vi "Handle Error.vi"(8 "error in (no error)":errorcluster, 11 "Guardian in":refnum<class "Guardian.lvclass">) -> (0 "error out":errorcluster, 2 "stop actor?":bool=TRUE, 3 "Guardian out":refnum<class "Guardian.lvclass">)   [LabVIEW 2026, in "TALOS.lvlib" / "Guardian.lvlib" / "Guardian.lvclass"]
doc: "This VI will process every error generated by a Guardian. If it is possible to solve it, log it in locale and not pass it to the Ancestor: otherwise, let it go, the Ancestor will try to do the same and, ultimately, it will push the error to the Error Manager of the Distributed System."
uses:
  Guardian.lvclass
  Ancestor/Ancestor/Ancestor.lvclass
  <vilib>/MultiError/TokenizeJSON/Multi Error Cluster.lvlib
  TALOS.lvlib
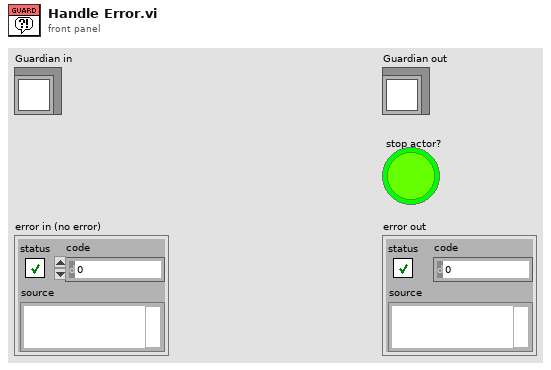
[diagram p1: front panel]
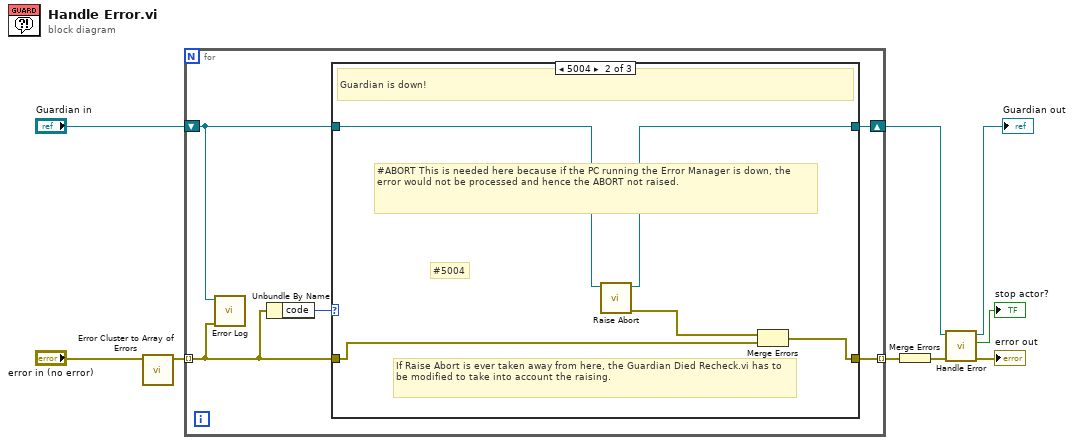
[diagram p0: block diagram]
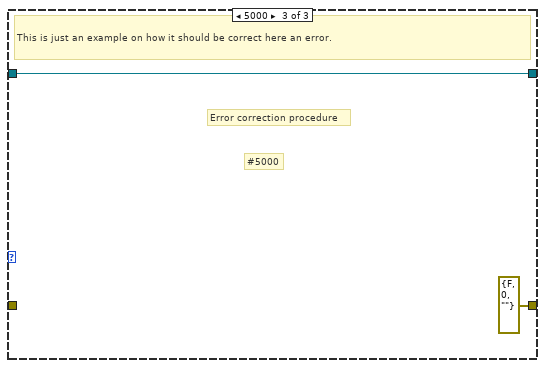
[diagram p3: hidden frame]
diagram:
  n1 = call <vilib>:"Error Cluster to Array of Errors.vi"("error"="error in (no error)") -> ("array of errors"=w2:errorcluster[])  [unwired: 10 in]
  n2 = for {
    tunnel: [w13] -> w4 mode=indexing
    tunnel: w2 -> [w11] mode=indexing
    shift-right: [w14] -> w5
    shift-left: "Guardian in" -> [w10]
    n3 = call "Error Log.vi"("error in (no error)"=w11, "Object in"=w10) -> ()  [unwired: 9 in, 1 out]
    n4 = Unbundle By Name(w11) -> ("code"=w12:i32)
    n5 = case shown="5004" w12 {
      tunnel: w10 -> [w16 w17 w23]
      tunnel: [w16 w18 w23] -> w14
      tunnel: w11 -> [w15 w21 _]
      tunnel: [w15 w20 errorcluster {"status"=FALSE, "code"=0, "source"=""} ("error IO")] -> w13
      frame Default {
        # "This error can't be handled by this Guardian alone: try with the Ancestor Handler and, ultimately, send it to the Error Manager of the Distributed system."
      }
      frame 5004 {
        # "If Raise Abort is ever taken away from here, the Guardian Died Recheck.vi has to be modified to take into account the raising."
        # "#5004"
        # "#ABORT This is needed here because if the PC running the Error Manager is down, the error would not be processed and hence the ABORT not raised."
        # "Guardian is down!"
        n6 = call "Raise Abort.vi"("Guardian in"=w17) -> ("error out"=w19:errorcluster, "Guardian out"=w18:refnum<class "Guardian.lvclass">)  [unwired: 9 in]
        n7 = Merge Errors(w19, w21) -> (w20:errorcluster)
      }
      frame 5000 {
        # "#5000"
        # "Error correction procedure"
        # "This is just an example on how it should be correct here an error."
      }
    }
  }
  n8 = Merge Errors(w4) -> (w1:errorcluster)
  n9 = call-parent "Handle Error.vi"("error in (no error)"=w1, "Ancestor in"=w5) -> ("error out"=→"error out":errorcluster, "stop actor?"=→"stop actor?":bool, "Ancestor out"=→"Guardian out":refnum<class "Guardian.lvclass">)  [unwired: 7 in]
